vi "EndTestSuite.vi"(8 "error in (no error)":errorcluster, 10 "TestSuite":refnum<class "TestSuite.lvclass">, 11 "TestListener in":refnum<class "TestListener.lvclass">) -> (0 "error out":errorcluster, 3 "TestListener out":refnum<class "TestListener.lvclass">)   [LabVIEW 2019, in "TestListener.lvclass"]
doc: "A test suite ended."
uses:
  TestListener.lvclass
  TestSuite/TestSuite.lvclass
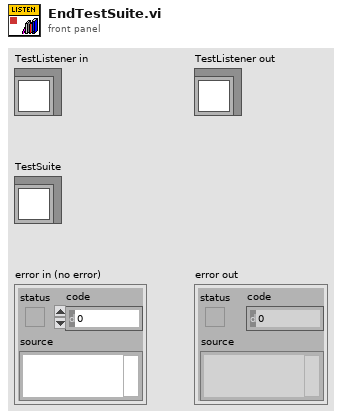
[diagram p1: front panel]
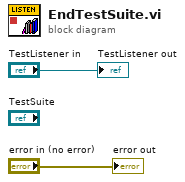
[diagram p0: block diagram]
diagram:
  "error out" <- "error in (no error)"
  "TestListener out" <- "TestListener in"
